vi "GetImageType.vi"(8 "error in (no error)":errorcluster, 11 "CameraDemo in":refnum<class "CameraDemo.lvclass">) -> (0 "error out":errorcluster, 2 "Image Type":u8 format="%.0x", 3 "CameraDemo out":refnum<class "CameraDemo.lvclass">)   [LabVIEW 2020, in "CameraI2COUSB.lvlib" / "CameraDemo.lvclass"]
uses:
  CameraDemo.lvclass
  CameraDemo.lvclass/CameraDemo.ctl
  Private/TypeDef/RegisterName.ctl
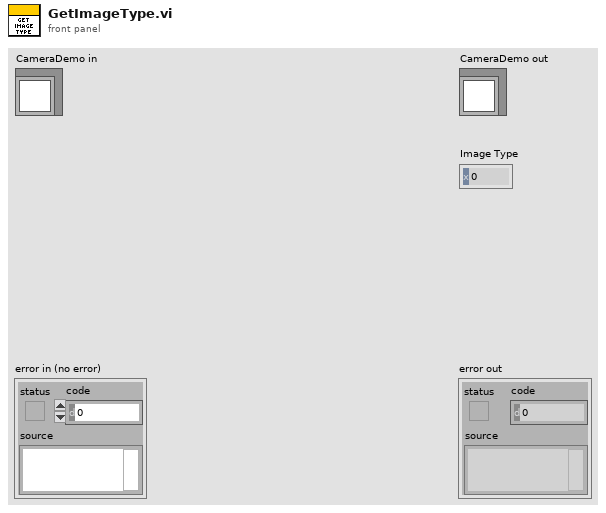
[diagram p1: front panel]
types:
  T1 = typedef "CameraI2COUSB.lvlib/CameraDemo.lvclass/RegisterName.ctl" = enum16{"Clock Rate", "Frame Rate", "Image Type", "Resolution", "Snap", "Start Streaming", "Stop Streaming"}
  T2 = typedef "CameraI2COUSB.lvlib/CameraDemo.lvclass/RegisterInfo.ctl" = cluster{"Address":u16, "Lenght":u32}
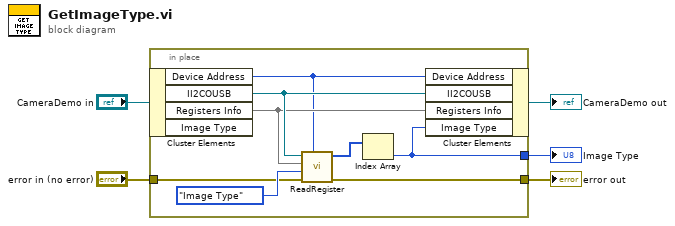
[diagram p0: block diagram]
diagram:
  n1 = in-place {
    in-place-border: "error in (no error)" -> [w9]
    in-place-border: [w8] -> w2
    in-place-border: [w6] -> w1
    n2 = in-place-cluster #1("CameraDemo in") -> ("Device Address"=w10:u8, "II2COUSB"=w13:refnum<class "II2COUSB.lvclass">, "Registers Info"=w12:map{T1, T2})  [unwired: 1 out]
    n3 = call "ReadRegister.vi"("Device Address"=w10, "error in (no error)"=w9, "Register Name"=RegisterName."Image Type", "Registers Info"=w12, "II2COUSB"=w13) -> ("error out"=w8:errorcluster, "DATA"=w7:u8[])  [unwired: 5 in]
    n4 = Index Array(array=w7) -> (element=w6:u8)  [unwired: 1 in]
    n5 = in-place-cluster #1("Device Address"=w10, "II2COUSB"=w13, "Registers Info"=w12, "Image Type"=w6) -> (→"CameraDemo out":refnum<class "CameraDemo.lvclass">)
  }
  "error out" <- w2
  "Image Type" <- w1
